vi "Read Macro Names.vi"(8 "error in (no error)":errorcluster, 11 "App Data Directory":path) -> (0 "error out":errorcluster, 3 "Macro Names":string[](array[string]))   [LabVIEW 2023]
doc: "Reads the list of macro names from <B>App Data Directory</B>."
uses:
  <userlib>/_OpenG.lib/file/file.llb/openg_file.lvlib
  <userlib>/_OpenG.lib/file/file.llb/Strip Path Extension - 1D Array of Strings__ogtk.vi
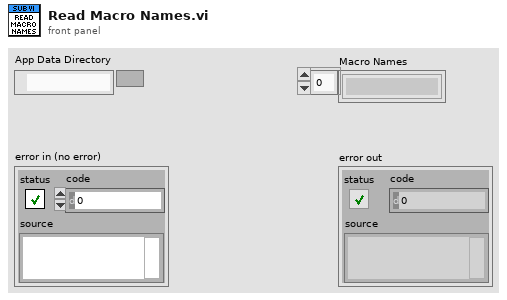
[diagram p1: front panel]
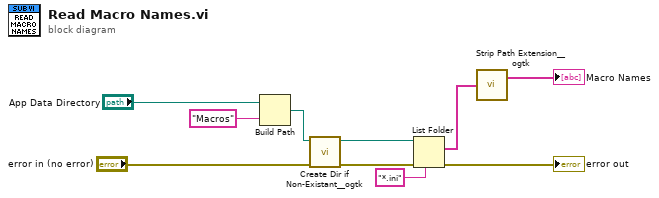
[diagram p0: block diagram]
diagram:
  n1 = Build Path(base path="App Data Directory", name or relative path="Macros" ("string")) -> (appended path=w6:path)
  n2 = call <userlib>:"Create Dir if Non-Existant__ogtk.vi"("error in (no error)"="error in (no error)", "Directory Path"=w6) -> ("error out"=w7:errorcluster, "dup Directory Path"=w5:path)  [unwired: 7 in, 1 out]
  n3 = List Folder(path=w5, pattern="*.ini", error in=w7) -> (filenames=w2:string[], error out=→"error out":errorcluster)  [unwired: 1 in, 2 out]
  n4 = call-poly <userlib>:"Strip Path Extension__ogtk.vi"("paths"=w2) -> ("roots"=→"Macro Names":string[])  [unwired: 1 out]
